vi "Actor Core.vi"(8 "error in":errorcluster, 11 "Pane Relief Main UI in":refnum<class "Pane Relief Main UI.lvclass">) -> (0 "error out":errorcluster, 3 "Actor out":refnum<class "Actor.lvclass">)   [LabVIEW 2015, in "Pane Relief Main UI.lvlib" / "Pane Relief Main UI.lvclass"]
uses:
  Pane Relief Main UI.lvclass
  <vilib>/ActorFramework/Actor/Actor.lvclass
  Pane Relief Main UI.lvclass/Pane Relief Main UI.ctl
  <vilib>/ActorFramework/Message Enqueuer/Message Enqueuer.lvclass/Message Enqueuer.ctl
  Pane Relief Main UI Messages/Select Panel Object Msg/Select Panel Object Msg.lvclass/Select Panel Object Msg.ctl
  Pane Relief Main UI Messages/Mouseover Panel Object Msg/Mouseover Panel Object Msg.lvclass/Mouseover Panel Object Msg.ctl
  <vilib>/ActorFramework/Message Enqueuer/Enqueue.vi
  <vilib>/ActorFramework/Message Priority Queue/Priority Enqueue.vi
  Pane Relief Main UI Messages/Rescale Msg/Rescale Msg.lvclass
  Pane Relief Main UI Messages/Select Panel Object Msg/Select Panel Object Msg.lvclass
  Pane Relief Main UI Messages/Mouseover Panel Object Msg/Mouseover Panel Object Msg.lvclass
  Pane Relief Main UI Messages/Refresh Msg/Refresh Msg.lvclass
  <vilib>/ActorFramework/Stop Msg/Stop Msg.lvclass
  <vilib>/MGI/Panel Manager/Panel Actor/Panel Actor/Panel Actor.lvclass
panel:
  out "Nav Pic":picture
  in  "Refresh Button":bool
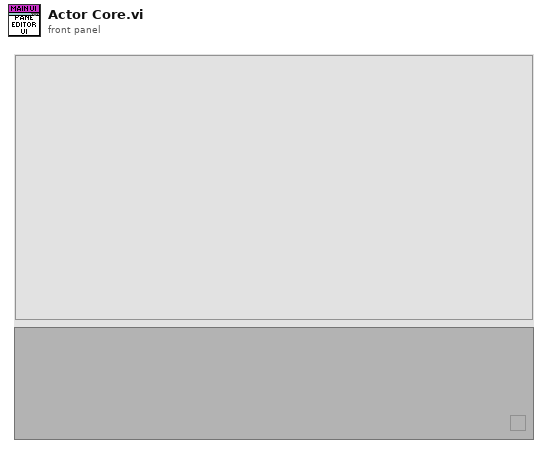
[diagram p1: front panel]
types:
  T1 = typedef "LVPoint32TypeDef.ctl" = cluster{"Horizontal":i32, "Vertical":i32}
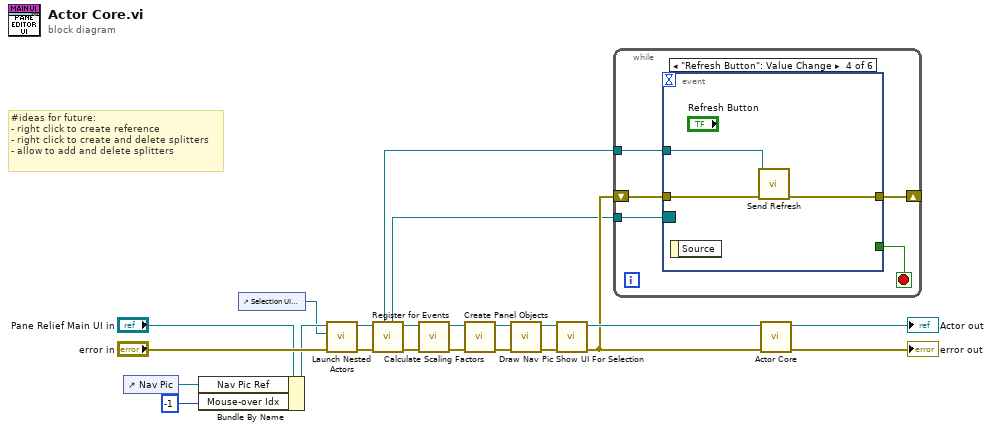
[diagram p0: block diagram]
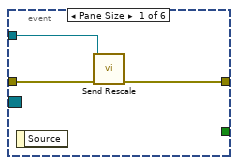
[diagram p2: hidden frame]
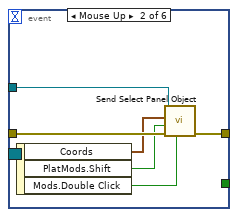
[diagram p3: hidden frame]
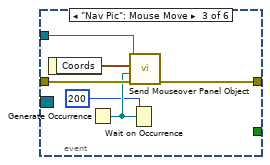
[diagram p4: hidden frame]
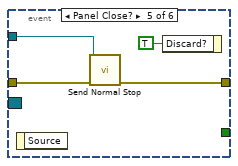
[diagram p5: hidden frame]
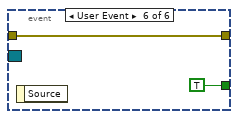
[diagram p6: hidden frame]
diagram:
  # "#ideas for future:\n- right click to create reference\n- right click to create and delete splitters\n- allow to add and delete splitters"
  n1 = control-ref of="Nav Pic"() -> (w19:refnum<vi>)
  n2 = Bundle By Name(cluster="Pane Relief Main UI in", "Nav Pic Ref"=w19, "Mouse-over Idx"=-1 ("UI Selections.Mouse-over Idx")) -> (w14:refnum<class "Pane Relief Main UI.lvclass">)
  n3 = control-ref of="Selection UI Subpanel"() -> (w13:refnum<vi>)
  n4 = call "Launch Nested Actors.vi"("error in (no error)"="error in", "Selection UI Subpanel Ref"=w13, "Pane Relief Main UI in"=w14) -> ("error out"=w12:errorcluster, "Pane Relief Main UI out"=w2:refnum<class "Pane Relief Main UI.lvclass">)  [unwired: 7 in]
  n5 = call <vilib>:"Register for Events.vi"("Error In"=w12, "Panel Actor in"=w2) -> ("Error Out"=w10:errorcluster, "Panel Actor out"=w1:refnum<class "Pane Relief Main UI.lvclass">, "Pnl Actor"=w11:refnum<event-registration>, "Self Enqueuer"=w3:refnum<class "Message Enqueuer.lvclass">)  [unwired: 6 in]
  n6 = call "Calculate Scaling Factors.vi"("error in (no error)"=w10, "Pane Relief Main UI in"=w1) -> ("error out"=w9:errorcluster, "Pane Relief Main UI out"=w6:refnum<class "Pane Relief Main UI.lvclass">)  [unwired: 8 in]
  n7 = call-dynamic "Create Panel Objects.vi"("Error In"=w9, "Pane Relief Main UI in"=w6) -> ("Error Out"=w8:errorcluster, "Pane Relief Main UI out"=w5:refnum<class "Pane Relief Main UI.lvclass">)  [unwired: 8 in]
  n8 = call-dynamic "Draw Nav Pic.vi"("Error In"=w8, "Pane Relief Main UI in"=w5) -> ("Error Out"=w7:errorcluster, "Pane Relief Main UI out"=w4:refnum<class "Pane Relief Main UI.lvclass">)  [unwired: 8 in]
  n9 = call-dynamic "Show UI For Selection.vi"("Error In"=w7, "Pane Relief Main UI in"=w4) -> ("Error Out"=w16:errorcluster, "Pane Relief Main UI out"=w17:refnum<class "Pane Relief Main UI.lvclass">)  [unwired: 8 in]
  n10 = while {
    shift-right: [w27] -> _
    shift-left: w16 -> [w25]
    tunnel: w3 -> [w26]
    tunnel: w11 -> [w24]
    stop <- w23 stop-if-true
    n11 = event shown="[3] \"Refresh Button\": Value Change" {
      selector: w24 -> [_ _ _ _ _ _]
      dyn-events: _ -> [_ _ _ _ _ _]
      timeout: _ -> [_ _ _ _ _ _]
      tunnel: [w29 w35 w40 w43 w48 w51] -> w27
      tunnel: w25 -> [w30 w36 w42 w44 w47 w51]
      tunnel: w26 -> [w28 w34 w39 w45 w49 _]
      tunnel: [_ _ _ _ _ TRUE] -> w23
      event Pane Size {
        n12 = event-data() -> ()  [unwired: 1 in, 1 out]
        n13 = call "Send Rescale.vi"("error in (no error)"=w30, "Message Enqueuer"=w28) -> ("error out"=w29:errorcluster)  [unwired: 8 in, 1 out]
      }
      event Mouse Up {
        n14 = event-data() -> ("Coords"=w33:T1, "PlatMods.Shift"=w32:bool, "Mods.Double Click"=w31:bool)  [unwired: 1 in]
        n15 = call "Send Select Panel Object.vi"("Select All Of Type"=w31, "error in (no error)"=w36, "Add To Selection"=w32, "Coords"=w33, "Message Enqueuer"=w34) -> ("error out"=w35:errorcluster)  [unwired: 5 in, 1 out]
      }
      event "Nav Pic": Mouse Move {
        n16 = event-data() -> ("Coords"=w41:T1)  [unwired: 1 in]
        n17 = Generate Occurrence() -> (w38:refnum<k4>)
        n18 = Wait on Occurrence(2:w38, 3:200 ("ms timeout (-1)")) -> ()  [unwired: 1 in, 1 out]
        n19 = call "Send Mouseover Panel Object.vi"("error in (no error)"=w42, "Occurrence"=w38, "Coords"=w41, "Message Enqueuer"=w39) -> ("error out"=w40:errorcluster)  [unwired: 6 in, 1 out]
      }
      event "Refresh Button": Value Change {
        n20 = event-data() -> ()  [unwired: 1 in, 1 out]
        n21 = call "Send Refresh.vi"("error in (no error)"=w44, "Message Enqueuer"=w45) -> ("error out"=w43:errorcluster)  [unwired: 8 in, 1 out]
      }
      event Panel Close? {
        n22 = event-data() -> ()  [unwired: 1 in, 1 out]
        n23 = call <vilib>:"Send Normal Stop.vi"("error in (no error)"=w47, "Message Enqueuer"=w49) -> ("error out"=w48:errorcluster)  [unwired: 9 in]
        n24 = event-data("Discard?"=TRUE) -> ()  [unwired: 1 in, 1 out]
      }
      event User Event {
        n25 = event-data() -> ()  [unwired: 1 in, 1 out]
      }
    }
  }
  n26 = call-parent "Actor Core.vi"("error in"=w16, "Panel Actor in"=w17) -> ("error out"=→"error out":errorcluster, "Actor out"=→"Actor out":refnum<class "Actor.lvclass">)  [unwired: 8 in]
